vi "Get Device by Type.vi"(7 "Device Type/Model":refnum<class "Device.lvclass">, 8 "error in (no error)":errorcluster, 11 "HAL Manager in":refnum<class "HAL Manager.lvclass">) -> (0 "error out":errorcluster, 2 "Device":refnum<class "Device.lvclass">, 3 "HAL Manager out":refnum<class "HAL Manager.lvclass">)   [LabVIEW 2020, in "HAL.lvlib" / "HAL Manager.lvclass"]
doc: "This VI is useful for simpler test applications where only a single device type is used. Without having to provide a specific name, this VI returns the first device matching the Type string returned by the passed in device type."
uses:
  HAL Manager.lvclass
  Device/Device.lvclass
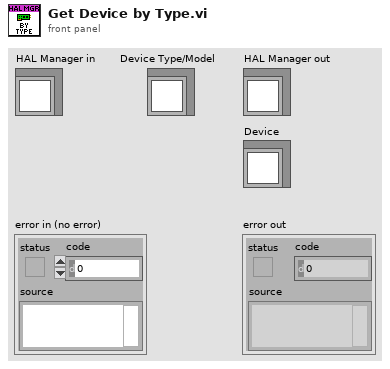
[diagram p1: front panel]
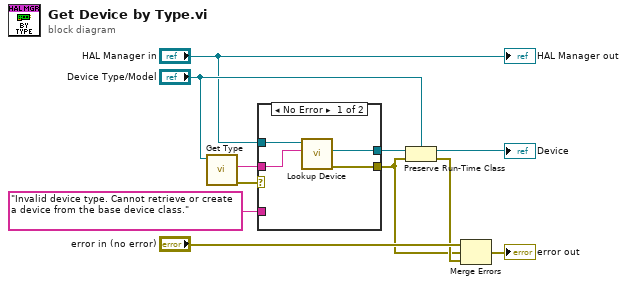
[diagram p0: block diagram]
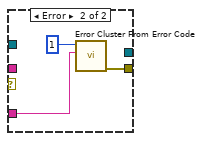
[diagram p2: hidden frame]
diagram:
  n1 = call-dynamic "Get Type.vi"("Device in"="Device Type/Model") -> ("error out"=w11:errorcluster, "Type"=w10:string)  [unwired: 8 in, 1 out]
  n2 = case shown="No Error" w11 {
    tunnel: w10 -> [w15 _]
    tunnel: "HAL Manager in" -> [w14 _]
    tunnel: [w12 w17] -> w2
    tunnel: [w13 _] -> w7
    tunnel: "Invalid device type. Cannot retrieve or create a device from the base device class." ("error message (\"\")") -> [_ w16]
    frame No Error {
      n3 = call "Lookup Device.vi"("Type"=w15, "HAL Manager in"=w14) -> ("error out"=w12:errorcluster, "Device"=w13:refnum<class "Device.lvclass">)  [unwired: 7 in, 1 out]
    }
    frame Error {
      n4 = call <vilib>:"Error Cluster From Error Code.vi"("error message (\"\")"=w16, "error code (0)"=1) -> ("error out"=w17:errorcluster)  [unwired: 7 in]
    }
  }
  n5 = Preserve Run-Time Class(object in=w7, error in=w2, 2:"Device Type/Model") -> (object out=→"Device":refnum<class "Device.lvclass">, error out=w3:errorcluster)
  n6 = Merge Errors("error in (no error)", w2, w3) -> (→"error out":errorcluster)
  "HAL Manager out" <- "HAL Manager in"
